vi "Fetch Multi Eval Meas SEM Trace Area Frequencies.vi"(6 "Area (1)":T2=1, 8 "error in (no error)":errorcluster, 9 "Offset Frequency (Positive)":T1=1 items=["Negative", "Positive"], 10 "Instance (1)":T3=1, 11 "VISA resource name":refnum<visa-resource-name>) -> (0 "error out":errorcluster, 1 "Frequencies":dbl[](array[numeric]) format="%^.3e", 2 "Reliability":i32, 3 "VISA resource name out":refnum<visa-resource-name>, 5 "Resolution BW":i32)   [LabVIEW 2020, in "Rohde&Schwarz CMWXP NR FR1 Measurement.lvlib"]
doc: "Returns the frequencies of a single spectrum emission mask area. The area is located below (negative) or above (positive) the carrier center frequency. At the returned frequencies, the power values are measured.\n\nAttributes:\nRSCMWXPNRFR1M_ATTR_FETCH_MULTI_EVAL_MEAS_SEM_TRACE_AREA_POSITIVE_FREQUENCIES\nRSCMWXPNRFR1M_ATTR_FETCH_MULTI_EVAL_MEAS_SEM_TRACE_AREA_NEGATIVE_FREQUENCIES\n\nRemote-control commands:\nFETCh:NRSub:MEAS<i>:MEValuation:TRACe:SEMask:AREA<area>:POSitive:FREQuency?\nFETCh:NRSub:MEAS<i>:MEValuation:TRACe:SEMask:AREA<area>:NEGative:FREQuency?"
uses:
  <instrlib>/Rohde&Schwarz CMWXP NR FR1 Measurement/Rohde&Schwarz CMWXP NR FR1 Measurement.lvlib
  <instrlib>/Rohde&Schwarz CMWXP NR FR1 Measurement/Private/_Instance.ctl
  <instrlib>/Rohde&Schwarz CMWXP NR FR1 Measurement/Private/_Area.ctl
  <instrlib>/Rohde&Schwarz CMWXP NR FR1 Measurement/Private/_Offset Frequency.ctl
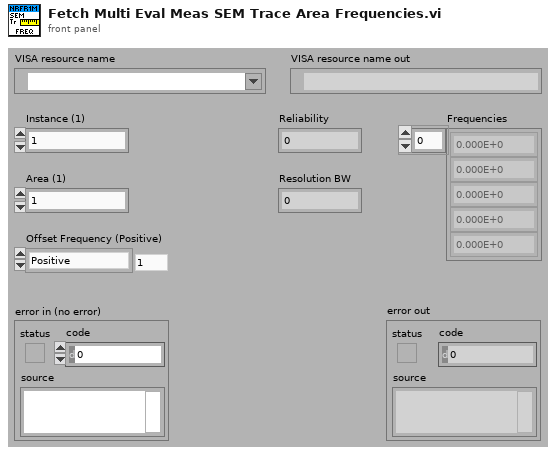
[diagram p1: front panel]
types:
  T1 = typedef "Rohde&Schwarz CMWXP NR FR1 Measurement.lvlib/_Offset Frequency.ctl" = i32
  T2 = typedef "Rohde&Schwarz CMWXP NR FR1 Measurement.lvlib/_Area.ctl" = i32
  T3 = typedef "Rohde&Schwarz CMWXP NR FR1 Measurement.lvlib/_Instance.ctl" = i32
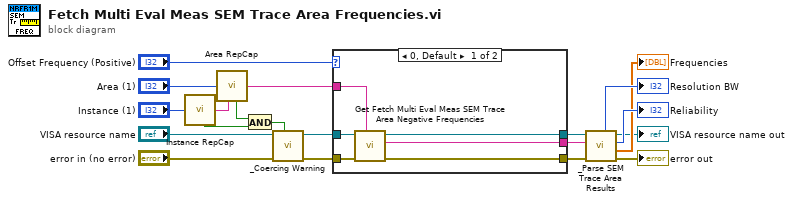
[diagram p0: block diagram]
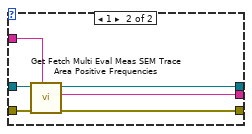
[diagram p2: hidden frame]
diagram:
  n1 = call <instrlib>:"Instance RepCap.vi"("Instance In"="Instance (1)") -> ("In Range?"=w15:bool, "RepCap Identifier Out"=w14:string)  [unwired: 1 in]
  n2 = call <instrlib>:"Area RepCap.vi"("SEM Area In"="Area (1)", "RepCap String In (\"\")"=w14) -> ("In Range?"=w13:bool, "RepCap Identifier Out"=w10:string)
  n3 = And(x=w13, y=w15) -> (x .and. y?=w18:bool)
  n4 = call <instrlib>:"_Coercing Warning.vi"("In Range?"=w18, "error in (no error)"="error in (no error)", "VISA resource name"="VISA resource name") -> ("error out"=w11:errorcluster, "VISA resource name out"=w12:refnum<visa-resource-name>)  [unwired: 7 in]
  n5 = case shown="0, Default" "Offset Frequency (Positive)" {
    tunnel: w12 -> [w26 w32]
    tunnel: w11 -> [w25 w31]
    tunnel: w10 -> [w24 w30]
    tunnel: [w23 w29] -> w6
    tunnel: [w22 w28] -> w7
    tunnel: [w21 w27] -> w8
    frame 0, Default {
      n6 = call "Get Fetch Multi Eval Meas SEM Trace Area Negative Frequencies"("Repeated Capabilities"=w24, "error in (no error)"=w25, "instrument handle"=w26) -> ("error out"=w21:errorcluster, "Fetch Multi Eval Meas SEM Trace Area Negative Frequencies"=w22:string, "instrument handle out"=w23:refnum<visa-resource-name>)  [unwired: 6 in]
    }
    frame 1 {
      n7 = call "Get Fetch Multi Eval Meas SEM Trace Area Positive Frequencies"("Repeated Capabilities"=w30, "error in (no error)"=w31, "instrument handle"=w32) -> ("error out"=w27:errorcluster, "Fetch Multi Eval Meas SEM Trace Area Positive Frequencies"=w28:string, "instrument handle out"=w29:refnum<visa-resource-name>)  [unwired: 6 in]
    }
  }
  n8 = call <instrlib>:"_Parse SEM Trace Area Results.vi"("error in (no error)"=w8, "Input String"=w7, "VISA resource name"=w6) -> ("error out"=→"error out":errorcluster, "Results"=→"Frequencies":dbl[], "Reliability"=→"Reliability":i32, "VISA resource name out"=→"VISA resource name out":refnum<visa-resource-name>, "Resolution BW"=→"Resolution BW":i32)  [unwired: 4 in]
